vi "nan_to_zero (SubVI).vi"(11 "Numeric in":dbl) -> (3 "Numeric out":dbl)   [LabVIEW 2018]
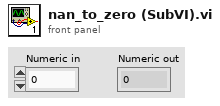
[diagram p1: front panel]
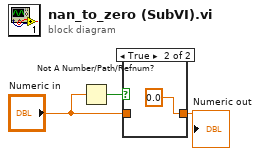
[diagram p0: block diagram]
diagram:
  n1 = Not A Number/Path/Refnum?(number/path/refnum="Numeric in") -> (NaN/Path/Refnum?=w1:bool)
  n2 = case shown="True" w1 {
    tunnel: [w4 0.0] -> w2
    tunnel: "Numeric in" -> [w4 _]
    frame False {
    }
    frame True {
    }
  }
  "Numeric out" <- w2
